vi "Get Industrial Controllers.vi"(8 "error in (no error)":errorcluster, 11 "Item Ref in":T1 format="%.0x") -> (0 "error out":errorcluster, 2 "Industrial Settings":T2 {"Write Refs"."Data Reference" format="%.0x"; "Read Refs"."Data Reference" format="%.0x"}, 3 "Device Ref out":T1 format="%.0x")   [LabVIEW 2019, in "Control Addon System Explorer.lvlib"]
uses:
  Control Addon System Explorer.lvlib
  <vilib>/NI VeriStand/Custom Device API/Custom Device Item Ref.ctl
  Addon Shared/Types/Compiled Industrial Settings.ctl
  <vilib>/NI VeriStand/Custom Device API/Block Data Reference.ctl
  <vilib>/NI VeriStand/Custom Device API/Data Reference.ctl
  Addon Shared/Types/Compiled Industrial Parameters.ctl
  <vilib>/NI VeriStand/Custom Device API/Data Access Type.ctl
  Types/Action.ctl
  Addon Shared/SubVIs/Constants.vi
  <vilib>/NI VeriStand/Custom Device Tools/Custom Device Utility Library/NI VeriStand - Search for All Items by GUID.vi
  <vilib>/NI VeriStand/Custom Device API/Get Item Property (Double).vi
  <vilib>/NI VeriStand/Custom Device API/Get Item Property (Boolean).vi
  <vilib>/NI VeriStand/Custom Device API/NI VeriStand - Set Item Property.vi
  <vilib>/NI VeriStand/Custom Device API/Set Item Property (Double).vi
  <vilib>/NI VeriStand/Custom Device API/Set Item Property (Boolean).vi
  <vilib>/NI VeriStand/Custom Device API/Get Item Property (Dependent Node Pointer).vi
  <vilib>/NI VeriStand/Custom Device Tools/Custom Device Utility Library/NI VeriStand - Search for Item by GUID.vi
  Addon Shared/Control Addon Shared.lvlib
  <vilib>/NI VeriStand/Custom Device API/Custom Device API.lvlib
  <vilib>/NI VeriStand/Custom Device Tools/Custom Device Utility Library/Custom Device Utility Library.lvlib
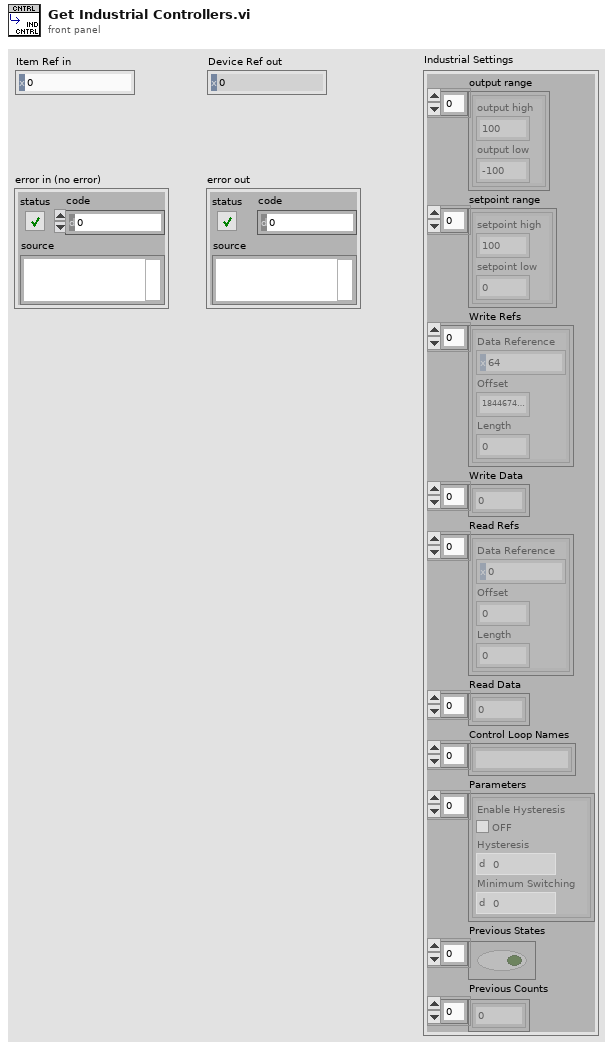
[diagram p1: front panel]
types:
  T1 = typedef "Custom Device API.lvlib/Custom Device Item Ref.ctl" = u64
  T2 = typedef "Control Addon Shared.lvlib/Compiled Industrial Settings.ctl" = cluster{"output range":cluster{"output high":dbl, "output low":dbl}[], "setpoint range":cluster{"setpoint high":dbl, "setpoint low":dbl}[], "Write Refs":T3[], "Write Data":dbl[], "Read Refs":T3[], "Read Data":dbl[], "Control Loop Names":string[], "Parameters":T5[], "Previous States":bool[], "Previous Counts":u64[]}
  T3 = typedef "Custom Device API.lvlib/Block Data Reference.ctl" = cluster{"Data Reference":T4, "Offset":u64, "Length":u64}
  T4 = typedef "Custom Device API.lvlib/Data Reference.ctl" = i32
  T5 = typedef "Control Addon Shared.lvlib/Compiled Industrial Parameters.ctl" = cluster{"Enable Hysteresis":bool, "Hysteresis":dbl, "Minimum Switching":u64}
  T6 = typedef "Custom Device API.lvlib/Data Access Type.ctl" = enum16{"Read", "Write"}
  T7 = typedef "Control Addon System Explorer.lvlib/Action.ctl" = enum16{"Get", "Set"}
  T8 = typedef "Custom Device API.lvlib/Custom Device Item Info.ctl" = cluster{"Name":string, "Is Channel":bool, "GUID":string, "Is Waveform":bool}
  T9 = typedef "Control Addon Shared.lvlib/Controller Settings.ctl" = cluster{"Output Max":dbl, "Output Min":dbl, "Setpoint Max":dbl, "Setpoint Min":dbl, "Use External Setpoint":bool, "Output Rate Limiter":dbl}
  T10 = typedef "Control Addon Shared.lvlib/Industrial Parameters.ctl" = cluster{"Enable Hysteresis":bool, "Hysteresis":dbl, "Enable Filter":bool, "Minimum Switching":dbl}
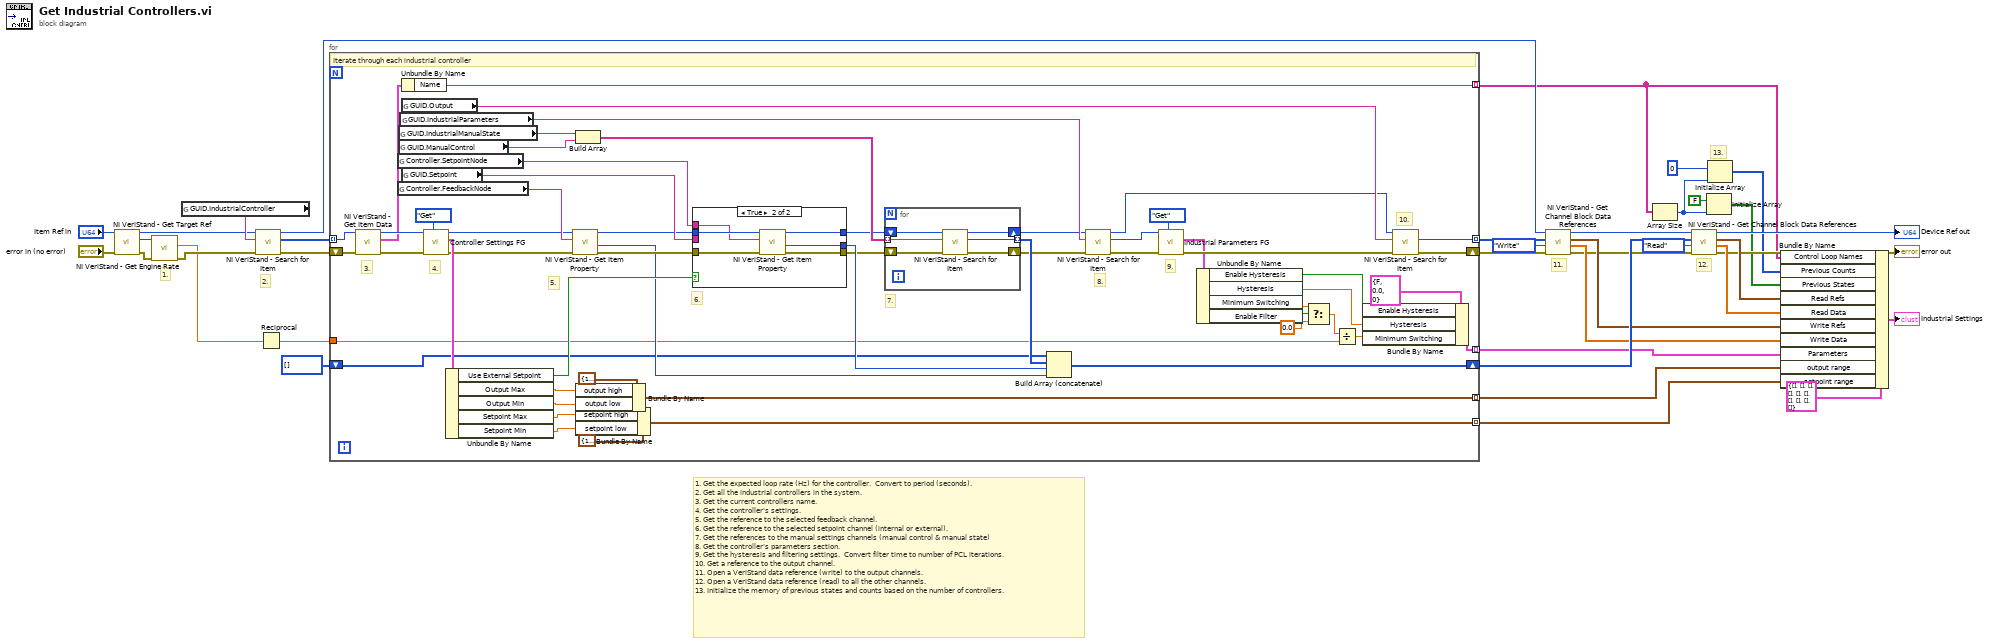
[diagram p0: block diagram]
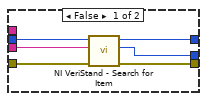
[diagram p2: hidden frame]
diagram:
  # "13."
  # "12."
  # "11."
  # "2."
  # "1."
  # "1. Get the expected loop rate (Hz) for the controller.  Convert to period (seconds).\n2. Get all the industrial controllers in the system.\n3. Get the current controllers name.\n4. Get the controller's settings.\n5. Get the reference to the selected feedback channel.\n6. Get the reference to the selected setpoint channel (internal or external).\n7. Get the references to the manual settings channels (manual control & manual state)\n8. Get the controller's parameters section.\n9. Get the hysteresis and filtering settings.  Convert filter time to number of PCL iterations.\n10. Get a reference to the output channel.\n11. Open a VeriStand data reference (write) to the output channels.\n12. Open a VeriStand data reference (read) to all the other channels. \n13. Initialize the memory of previous states and counts based on the number of controllers."
  n1 = call <vilib>:"NI VeriStand - Get Target Ref.vi"("error in"="error in (no error)", "Item Ref in"="Item Ref in") -> ("error out"=w2:errorcluster, "Target Ref"=w4:T1, "Item Ref out"=w3:T1)  [unwired: 6 in, 1 out]
  n2 = call <vilib>:"NI VeriStand - Get Engine Rate.vi"("error in (no error)"=w2, "Item Ref in"=w4) -> ("error out"=w11:errorcluster, "Rate (Hz)"=w5:dbl)  [unwired: 7 in, 1 out]
  n3 = global read "Constants.vi" "GUID.IndustrialController"() -> (w36:string)
  n4 = call-poly <vilib>:"NI VeriStand - Search for Item.vi"("error in"=w11, "Item GUID"=w36, "Section Ref in"=w3) -> ("error out"=w33:errorcluster, "Item Refs"=w35:T1[], "Section Ref out"=w34:T1)  [unwired: 5 in, 1 out]
  n5 = Reciprocal(x=w5) -> (1/x=w9:dbl)
  n6 = for {
    shift-right: [w62] -> w16
    shift-left: w33 -> [w53]
    tunnel: w35 -> [w55] mode=indexing
    tunnel: [w61] -> w29 mode=indexing
    tunnel: [w60] -> w28 mode=indexing
    tunnel: [w59] -> w19 mode=indexing
    tunnel: [w44] -> w15 mode=indexing
    shift-right: [w58] -> w31
    shift-left: T1[] [] -> [w56]
    tunnel: [w50] -> w13 mode=indexing
    tunnel: w9 -> [w42]
    # "10."
    # "9."
    # "8."
    # "7."
    # "6."
    # "5."
    # "4."
    # "3."
    # "Iterate through each industrial controller"
    n7 = call <vilib>:"NI VeriStand - Get Item Data.vi"("error in (no error)"=w53, "Item Ref in"=w55) -> ("error out"=w52:errorcluster, "Item Info"=w51:T8, "Item Ref out"=w54:T1)  [unwired: 6 in, 1 out]
    n8 = global read "Constants.vi" "Controller.SetpointNode"() -> (w91:string)
    n9 = global read "Constants.vi" "Controller.FeedbackNode"() -> (w90:string)
    n10 = global read "Constants.vi" "GUID.IndustrialManualState"() -> (w87:string)
    n11 = global read "Constants.vi" "GUID.ManualControl"() -> (w82:string)
    n12 = global read "Constants.vi" "GUID.IndustrialParameters"() -> (w84:string)
    n13 = Unbundle By Name(w51) -> ("Name"=w50:string)
    n14 = global read "Constants.vi" "GUID.Output"() -> (w80:string)
    n15 = global read "Constants.vi" "GUID.Setpoint"() -> (w89:string)
    n16 = call "Controller Settings FG.vi"("Action"=Action."Get", "error in (no error)"=w52, "Node Ptr"=w54) -> ("error out"=w68:errorcluster, "Controller Settings"=w76:T9, "Item Ref out"=w67:T1)  [unwired: 6 in]
    n17 = Unbundle By Name(w76) -> ("Use External Setpoint"=w92:bool, "Output Max"=w70:dbl, "Output Min"=w71:dbl, "Setpoint Max"=w72:dbl, "Setpoint Min"=w73:dbl)
    n18 = call-poly <vilib>:"NI VeriStand - Get Item Property.vi"("error in (no error)"=w68, "Property Name"=w90, "Item Ref in"=w67) -> ("error out"=w65:errorcluster, "Dependent Node Ref"=w57:T1, "Item Ref out"=w66:T1)  [unwired: 5 in, 1 out]
    n19 = Build Array(w87, w82) -> (w88:string[])
    n20 = Bundle By Name(cluster=cluster{"output high":dbl, "output low":dbl} {"output high"=100.0, "output low"=-100.0} ("output range"), "output high"=w70, "output low"=w71) -> (w60:cluster{"output high":dbl, "output low":dbl})
    n21 = Bundle By Name(cluster=cluster{"setpoint high":dbl, "setpoint low":dbl} {"setpoint high"=100.0, "setpoint low"=0.0} ("setpoint range"), "setpoint high"=w72, "setpoint low"=w73) -> (w61:cluster{"setpoint high":dbl, "setpoint low":dbl})
    n22 = case shown="True" w92 {
      tunnel: w65 -> [w105 w111]
      tunnel: w66 -> [w102 w110]
      tunnel: [w104 w109] -> w64
      tunnel: [w103 w108] -> w63
      tunnel: w91 -> [_ w107]
      tunnel: [w100 w106] -> w69
      tunnel: w89 -> [w101 _]
      frame False {
        n23 = call-poly <vilib>:"NI VeriStand - Search for Item.vi"("error in"=w105, "Item GUID"=w101, "Section Ref in"=w102) -> ("error out"=w104:errorcluster, "Item Ref"=w100:T1, "Section Ref out"=w103:T1)  [unwired: 5 in, 1 out]
      }
      frame True {
        n24 = call-poly <vilib>:"NI VeriStand - Get Item Property.vi"("error in (no error)"=w111, "Property Name"=w107, "Item Ref in"=w110) -> ("error out"=w109:errorcluster, "Dependent Node Ref"=w106:T1, "Item Ref out"=w108:T1)  [unwired: 5 in, 1 out]
      }
    }
    n25 = for {
      shift-right: [w95] -> w79
      shift-left: w64 -> [w99]
      shift-right: [w97] -> w78
      shift-left: w63 -> [w98]
      tunnel: w88 -> [w96] mode=indexing
      tunnel: [w94] -> w81 mode=indexing
      n26 = call-poly <vilib>:"NI VeriStand - Search for Item.vi"("error in"=w99, "Item GUID"=w96, "Section Ref in"=w98) -> ("error out"=w95:errorcluster, "Item Ref"=w94:T1, "Section Ref out"=w97:T1)  [unwired: 5 in, 1 out]
    }
    n27 = Build Array (concatenate)(w56, w81, w69, w57) -> (w58:T1[])
    n28 = call-poly <vilib>:"NI VeriStand - Search for Item.vi"("error in"=w79, "Item GUID"=w84, "Section Ref in"=w78) -> ("error out"=w86:errorcluster, "Item Ref"=w85:T1, "Section Ref out"=w77:T1)  [unwired: 5 in, 1 out]
    n29 = call "Industrial Parameters FG.vi"("Action"=Action."Get", "error in (no error)"=w86, "Node Ptr"=w85) -> ("error out"=w49:errorcluster, "Parameters"=w45:T10)  [unwired: 6 in, 1 out]
    n30 = Unbundle By Name(w45) -> ("Enable Hysteresis"=w39:bool, "Hysteresis"=w38:dbl, "Minimum Switching"=w47:dbl, "Enable Filter"=w48:bool)
    n31 = Select(t=w47, s=w48, f=0.0) -> (s? t:f=w43:dbl)
    n32 = Divide(x=w43, y=w42) -> (x/y=w41:dbl)
    n33 = Bundle By Name(cluster=T5 {"Enable Hysteresis"=FALSE, "Hysteresis"=0.0, "Minimum Switching"=0} ("Parameters"), "Enable Hysteresis"=w39, "Hysteresis"=w38, "Minimum Switching"=w41) -> (w44:T5)
    n34 = call-poly <vilib>:"NI VeriStand - Search for Item.vi"("error in"=w49, "Item GUID"=w80, "Section Ref in"=w77) -> ("error out"=w62:errorcluster, "Item Ref"=w59:T1)  [unwired: 5 in, 2 out]
  }
  n35 = call <vilib>:"NI VeriStand - Get Channel Block Data References.vi"("error in (no error)"=w16, "Access"=Data_Access_Type."Write", "Channel Refs"=w19, "Device Ref in"=w34) -> ("error out"=w17:errorcluster, "Values Array"=w27:dbl[], "Block Data Refs"=w26:T3[], "Device Ref out"=w20:T1)  [unwired: 4 in]
  n36 = Array Size(array=w13) -> (size(s)=w8:i32)
  n37 = call <vilib>:"NI VeriStand - Get Channel Block Data References.vi"("error in (no error)"=w17, "Access"=Data_Access_Type."Read", "Channel Refs"=w31, "Device Ref in"=w20) -> ("error out"=→"error out":errorcluster, "Values Array"=w25:dbl[], "Block Data Refs"=w24:T3[], "Device Ref out"=→"Device Ref out":T1)  [unwired: 4 in]
  n38 = Initialize Array(FALSE, w8) -> (w12:bool[])
  n39 = Initialize Array(u64 0, w8) -> (w6:u64[])
  n40 = Bundle By Name(cluster=T2 {"output range"=[], "setpoint range"=[], "Write Refs"=[], "Write Data"=[], "Read Refs"=[], "Read Data"=[], "Control Loop Names"=[], "Parameters"=[], "Previous States"=[], "Previous Counts"=[]} ("PID Settings"), "Control Loop Names"=w13, "Previous Counts"=w6, "Previous States"=w12, "Read Refs"=w24, "Read Data"=w25, "Write Refs"=w26, "Write Data"=w27, "Parameters"=w15, "output range"=w28, "setpoint range"=w29) -> (→"Industrial Settings":T2)
